vi "Init Select Module Ring.vi"(8 "error in":errorcluster, 11 "Select Module Ring Ref":refnum<vi>) -> (0 "error out":errorcluster, 1 "Module Ring Value":i32=-1, 3 "Value for All Modules":i32)   [LabVIEW 2023, in "Tree Handlr.lvlib"]
doc: "Initialize the strings and values in the module selector ring.\n_____\nBased on DQMH Project Template 7.0.1.1316."
uses:
  Tree Handlr.lvlib
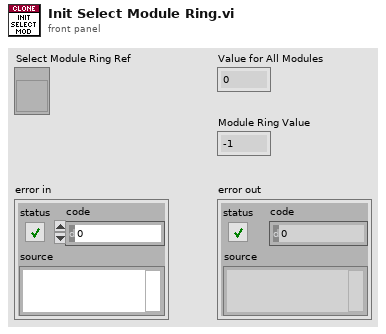
[diagram p1: front panel]
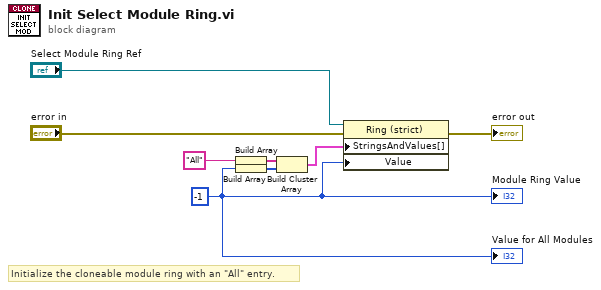
[diagram p0: block diagram]
diagram:
  w8 = -1 ("element")
  # "Initialize the cloneable module ring with an \"All\" entry."
  n1 = Build Array("All" ("element")) -> (w6:string[])
  n2 = Build Array(w8) -> (w7:i32[])
  n3 = Build Cluster Array(w6, w7) -> (w1:cluster{"element":string, "element":i32}[])
  n4 = property on="Property Node" class="Ring (strict)"(reference="Select Module Ring Ref", error in="error in", "StringsAndValues[]"=w1, "Value"=w8) -> (error out=→"error out":errorcluster)  [unwired: 1 out]
  "Value for All Modules" <- w8
  "Module Ring Value" <- w8
